vi "VariantAndNameArrayToArrays.vi"(1 "Names Array":string[](array[string]), 4 "Variant Array":variant[](array[variant])) -> (14 "bool":bool[](array[boolean]), 15 "boolNames":string[](array[string]), 16 "num":dbl[](array[numeric]), 17 "numNames":string[](array[string]), 18 "string":string[](array[string]), 19 "stringNames":string[](array[string]))   [LabVIEW 2019]
uses:
  <vilib>/Utility/Data Type/Type Definitions/Data Type.ctl
  <vilib>/Utility/Data Type/NI_Data Type.lvlib
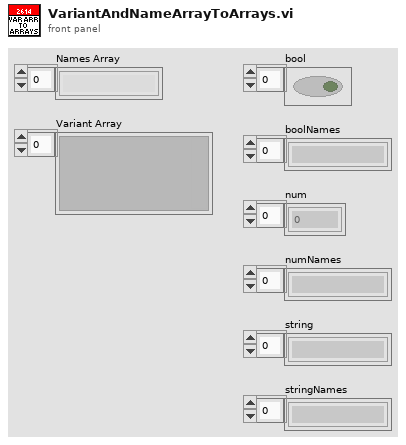
[diagram p1: front panel]
types:
  T1 = typedef "NI_Data Type.lvlib/Data Type.ctl" = enum8{"Invalid Type", "Void", "I8", "I16", "I32", "I64", "U8", "U16", "U32", "U64", "Single Float", "Double Float", "Extended Float", "Single Complex", "Double Complex", "Extended Complex", "Enum U8", "Enum U16", "Enum U32", "Enum U64", "Single Float With Unit", "Double Float With Unit", "Extended Float With Unit", "Single Complex with Unit", "Double Complex with Unit", "Extended Complex with Unit", "Boolean", "String", "Path", "Picture", "Tag", "Array", "Cluster", "Variant", "LV Variant", "Waveform", "Timestamp", "Digital Waveform", "Digital Data", "ExpressData", "Refnum", "External Data", "VI", "Poly VI", "LabVIEW Class Instance", "Fixed Point", "Set Collection", "Map Collection"}
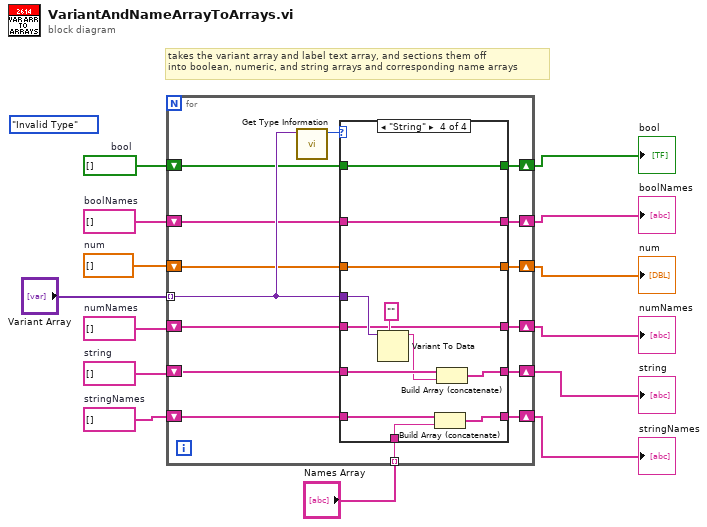
[diagram p0: block diagram]
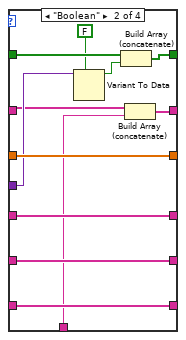
[diagram p3: hidden frame]
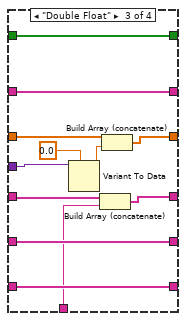
[diagram p4: hidden frame]
diagram:
  (unwired) Data_Type."Invalid Type" ("type")
  w5 = string[] []  # boolNames
  w6 = string[] []  # numNames
  w7 = string[] []  # stringNames
  w4 = bool[] []  # bool
  w3 = dbl[] []  # num
  w2 = string[] []  # string
  # "takes the variant array and label text array, and sections them off \ninto boolean, numeric, and string arrays and corresponding name arrays"
  n1 = for {
    tunnel: "Variant Array" -> [w28] mode=indexing
    shift-right: [w26] -> w12
    shift-left: w2 -> [w27]
    shift-right: [w23] -> w9
    shift-left: w4 -> [w24]
    shift-right: [w22] -> w14
    shift-left: w3 -> [w25]
    shift-right: [w19] -> w13
    shift-left: w7 -> [w21]
    shift-right: [w17] -> w11
    shift-left: w6 -> [w18]
    shift-right: [w15] -> w10
    shift-left: w5 -> [w16]
    tunnel: "Names Array" -> [w20] mode=indexing
    n2 = call <vilib>:"Get Type Information.vi"("variant"=w28) -> ("type"=w29:T1)  [unwired: 6 in, 4 out]
    n3 = case shown="\"String\"" w29 {
      tunnel: w28 -> [_ w43 w57 w71]
      tunnel: w27 -> [w35 w46 w58 w69]
      tunnel: [w35 w46 w58 w67] -> w26
      tunnel: w25 -> [w34 w47 w55 w66]
      tunnel: w24 -> [w33 w44 w59 w65]
      tunnel: [w33 w41 w59 w65] -> w23
      tunnel: [w34 w47 w53 w66] -> w22
      tunnel: w21 -> [w30 w39 w52 w64]
      tunnel: w20 -> [_ w37 w49 w62]
      tunnel: [w30 w39 w52 w63] -> w19
      tunnel: w18 -> [w31 w38 w50 w61]
      tunnel: [w31 w38 w48 w61] -> w17
      tunnel: w16 -> [w32 w40 w51 w60]
      tunnel: [w32 w36 w51 w60] -> w15
      frame "Invalid Type", Default {
      }
      frame "Boolean" {
        n4 = Variant To Data(type=FALSE, Variant=w43) -> (data=w45:bool)  [unwired: 1 in, 1 out]
        n5 = Build Array (concatenate)(w44, w45) -> (w41:bool[])
        n6 = Build Array (concatenate)(w40, w37) -> (w36:string[])
      }
      frame "Double Float" {
        n7 = Variant To Data(type=0.0, Variant=w57) -> (data=w54:dbl)  [unwired: 1 in, 1 out]
        n8 = Build Array (concatenate)(w50, w49) -> (w48:string[])
        n9 = Build Array (concatenate)(w55, w54) -> (w53:dbl[])
      }
      frame "String" {
        n10 = Variant To Data(type="", Variant=w71) -> (data=w68:string)  [unwired: 1 in, 1 out]
        n11 = Build Array (concatenate)(w64, w62) -> (w63:string[])
        n12 = Build Array (concatenate)(w69, w68) -> (w67:string[])
      }
    }
  }
  "num" <- w14
  "stringNames" <- w13
  "string" <- w12
  "numNames" <- w11
  "boolNames" <- w10
  "bool" <- w9
